vi "GenericIMAQGetConfig.vi"(10 "Camera (in)":T1={"Framerate (Hz)"=100, "Exposure time (us)"=100, "Image size"={"Width"=1280, "Height"=1024}, "Number of buffers"=30}, 11 "IMAQ Refnum in":refnum<k11>) -> (2 "Camera":T1={"Framerate (Hz)"=100, "Exposure time (us)"=100, "Image size"={"Width"=1280, "Height"=1024}, "Number of buffers"=30}, 3 "IMAQ Session Out":refnum<k11>)   [LabVIEW 2011]
uses:
  Main/Camera/GenericCameraConfigType.ctl
  Global_GenericIMAQCamera_HardwareConfig.vi
panel:
  out "framerate":i32
  out "Exposure Time (us)":i32
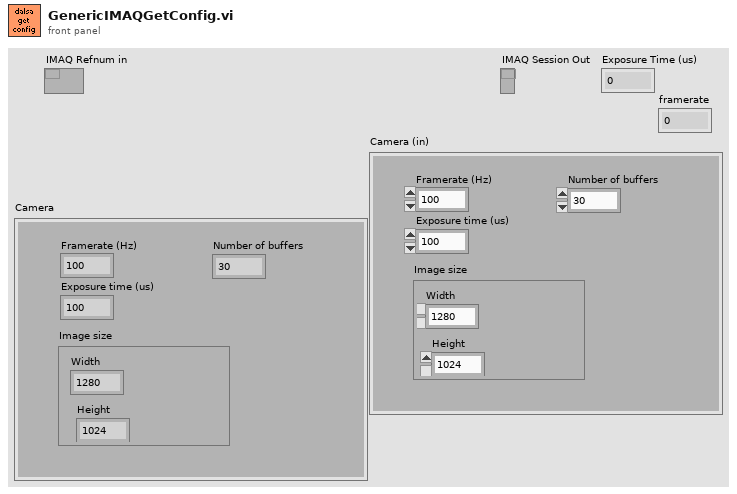
[diagram p1: front panel]
types:
  T1 = typedef "GenericCameraConfigType.ctl" = cluster{"Framerate (Hz)":i32, "Exposure time (us)":i32, "Image size":cluster{"Width":i32, "Height":i32}, "Number of buffers":i32}
  T2 = typedef "GenericIMAQHardwareConfig.ctl" = cluster{"Camera config mode":enum16{"Serial", "IMAQParam", "NoConfig"}, "Frame rate set cmd":string, "Exposure time set cmd":string, "Frame rate get cmd":string, "Exposure time get cmd":string, "IMAQ Identifier":string, "Serial return skip chars":i32, "Set width/height":string, "Set offset xy":string, "Get width":string, "Get height":string, "Get offset X":string, "Get offset Y":string, "Full frame size":cluster{"width":i32, "height":i32}}
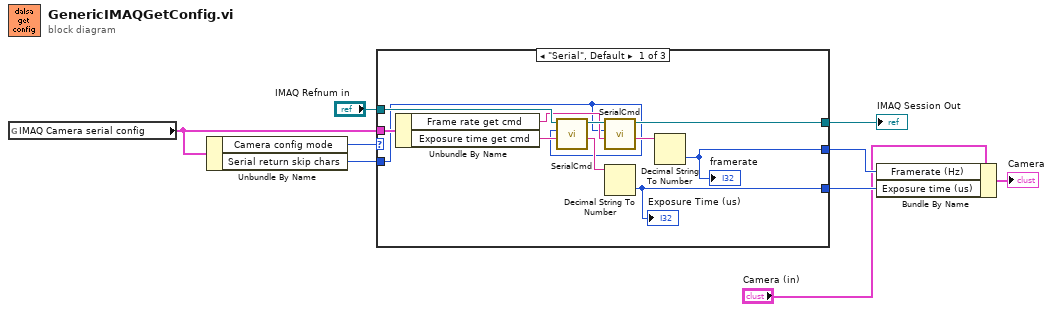
[diagram p0: block diagram]
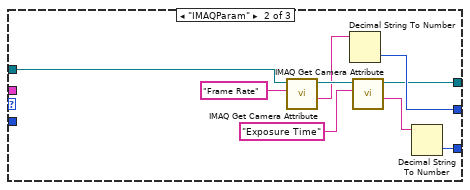
[diagram p2: hidden frame]
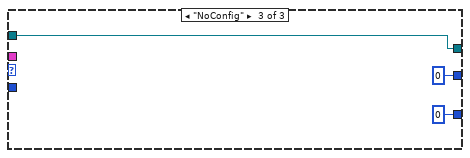
[diagram p3: hidden frame]
diagram:
  n1 = global read "Global_GenericIMAQCamera_HardwareConfig.vi" "IMAQ Camera serial config"() -> (w2:T2)
  n2 = Unbundle By Name(w2) -> ("Camera config mode"=w3:enum16{"Serial", "IMAQParam", "NoConfig"}, "Serial return skip chars"=w1:i32)
  n3 = case shown="\"Serial\", Default" w3 {
    tunnel: "IMAQ Refnum in" -> [w20 w21 w32]
    tunnel: [w19 w23 0] -> w8
    tunnel: [w18 w25 0] -> w7
    tunnel: [w14 w22 w32] -> w4
    tunnel: w2 -> [w13 _ _]
    tunnel: w1 -> [w10 _ _]
    frame "Serial", Default {
      n4 = Unbundle By Name(w13) -> ("Frame rate get cmd"=w11:string, "Exposure time get cmd"=w12:string)
      n5 = call "SerialCmd.vi"("command"=w12, "Return string skip chars (2)"=w10, "IMAQ Refnum in"=w20) -> ("String Read"=w16:string, "IMAQ Session Out"=w17:refnum<k11>)  [unwired: 5 in, 2 out]
      n6 = call "SerialCmd.vi"("command"=w11, "Return string skip chars (2)"=w10, "IMAQ Refnum in"=w17) -> ("String Read"=w15:string, "IMAQ Session Out"=w14:refnum<k11>)  [unwired: 5 in, 2 out]
      n7 = Decimal String To Number(string=w16) -> (number=w18:i32)  [unwired: 2 in, 1 out]
      "Exposure Time (us)" <- w18
      n8 = Decimal String To Number(string=w15) -> (number=w19:i32)  [unwired: 2 in, 1 out]
      "framerate" <- w19
    }
    frame "IMAQParam" {
      n9 = call <vilib>:"IMAQ Get Camera Attribute.vi"("Camera Attribute"="Frame Rate", "IMAQ Session In"=w21) -> ("Attribute Value"=w24:string, "IMAQ Session Out"=w29:refnum<k11>)  [unwired: 5 in, 1 out]
      n10 = Decimal String To Number(string=w24) -> (number=w23:i32)  [unwired: 2 in, 1 out]
      n11 = call <vilib>:"IMAQ Get Camera Attribute.vi"("Camera Attribute"="Exposure Time", "IMAQ Session In"=w29) -> ("Attribute Value"=w26:string, "IMAQ Session Out"=w22:refnum<k11>)  [unwired: 5 in, 1 out]
      n12 = Decimal String To Number(string=w26) -> (number=w25:i32)  [unwired: 2 in, 1 out]
    }
    frame "NoConfig" {
    }
  }
  "IMAQ Session Out" <- w4
  n13 = Bundle By Name(cluster="Camera (in)", "Framerate (Hz)"=w8, "Exposure time (us)"=w7) -> (→"Camera":T1)
